vi "Stop Module.vi"(6 "Timeout to Wait for Stop (s) (-1: no timeout)":dbl=-1.0, 8 "error in":errorcluster, 9 "Wait for Module to Stop? (F)":bool, 10 "Origin":string) -> (0 "error out":errorcluster)   [LabVIEW 2025, in "CML UI.lvlib"]
doc: "Send the Stop request to the Module's Main.vi.\n\nIf <b>Wait for Module to Stop?</b> is TRUE, this VI will wait until the module main VI stops, and will timeout at the <b>Timeout to Wait for Stop</b> value. This value defaults to \"-1\", which means the VI will not timeout, and will always wait until the module main VI stops before completing execution.\n\nNote: The <b>Timeout to Wait for Stop</b> value is ignored if 'Wait for Module to Stop?' is set to FALSE.\n_____\nBased on DQMH Project Template 4.0.0.47.\n\n<b>Note:</b> This VI was modified by the <b>Validate DQMH Module</b> tool to add calls to the Semaphore VIs to synchronize actions between the Start Module and Stop Module VIs.\n_____\nBased on DQMH Dev Tools: Project Template 7.1.0.1503."
uses:
  CML UI.lvlib
  Stop Argument--cluster.ctl
  <vilib>/event_ctls.llb/usereventprio.ctl
panel:
  # "Note: The 'Timeout to Wait for Stop' value is ignored if 'Wait for Module to Stop?' is set to FALSE."
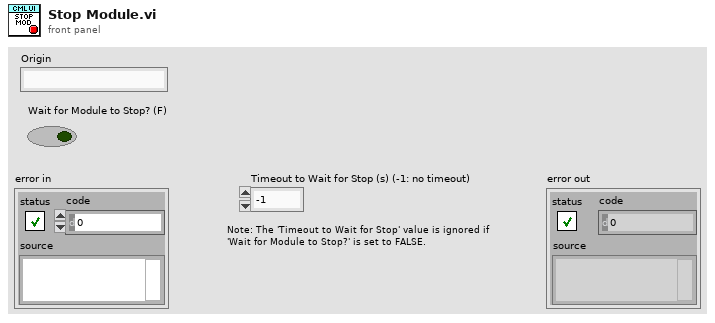
[diagram p1: front panel]
types:
  T1 = typedef "CML UI.lvlib/Stop Argument--cluster.ctl" = cluster{"Origin":string, "Exit via Stop Module Req?":bool, "Wait for Module to stop?":bool}
  T2 = typedef "usereventprio.ctl" = enum32{"high priority", "normal priority"}
  T3 = typedef "CML UI.lvlib/Request Events--cluster.ctl" = cluster{"Stop Module":refnum<user-event>, "Show Panel":refnum<user-event>, "Hide Panel":refnum<user-event>, "Get Module Execution Status":refnum<user-event>, "Show Diagram":refnum<user-event>}
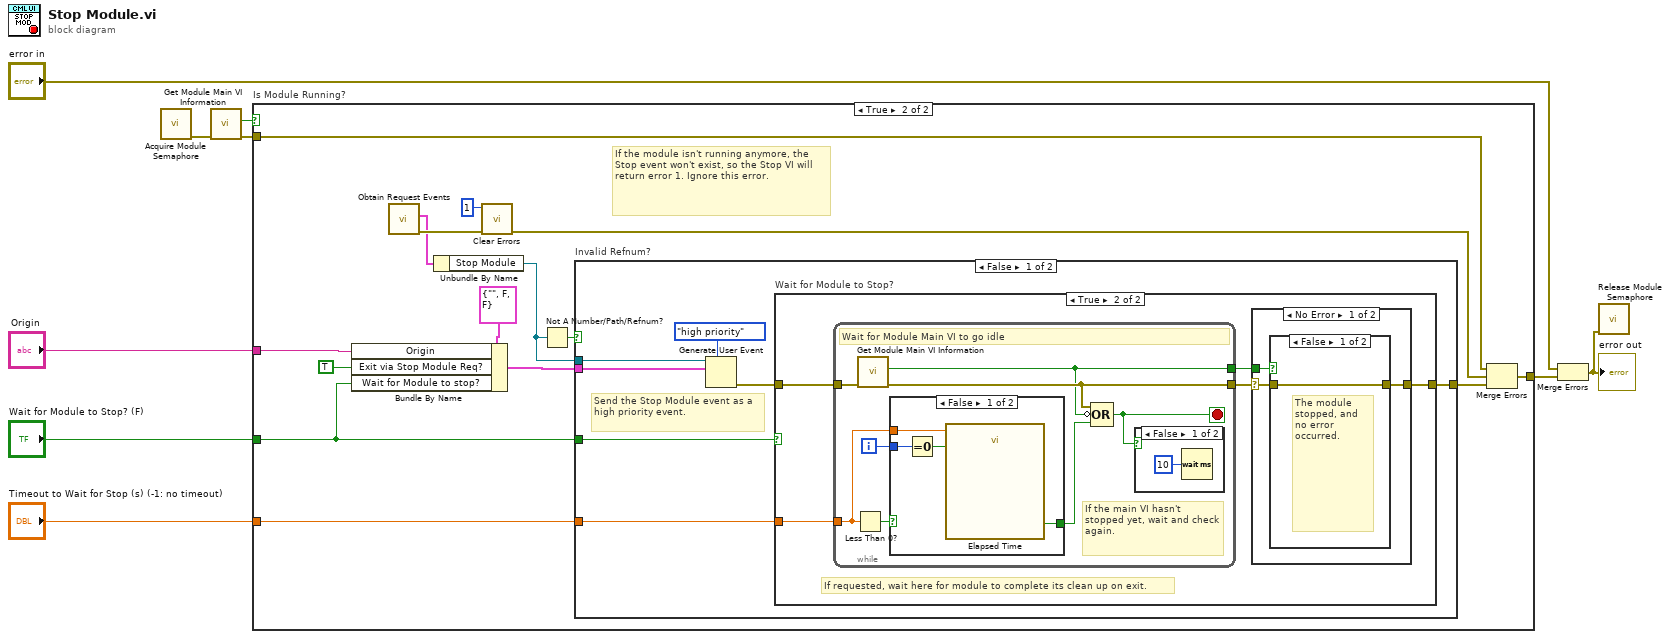
[diagram p0: block diagram]
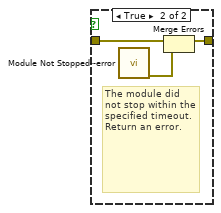
[diagram p4: hidden frame]
diagram:
  n1 = call "Acquire Module Semaphore.vi"() -> ("error out"=w1:errorcluster)  [unwired: 11 in]
  n2 = call "Get Module Main VI Information.vi"("error in"=w1) -> ("error out"=w6:errorcluster, "Is Module Running?"=w5:bool)  [unwired: 7 in, 2 out]
  n3 = case "Is Module Running?" shown="True" w5 {
    tunnel: [w10 w24] -> w9
    tunnel: "Origin" -> [_ w23]
    tunnel: w6 -> [w10 w15]
    tunnel: "Wait for Module to Stop? (F)" -> [_ w12]
    tunnel: "Timeout to Wait for Stop (s) (-1: no timeout)" -> [_ w11]
    frame False {
      # "The module is not running, there is no need to run the Stop Module code."
    }
    frame True {
      # "If the module isn't running anymore, the Stop event won't exist, so the Stop VI will return error 1. Ignore this error."
      n4 = Bundle By Name(cluster=T1 {"Origin"="", "Exit via Stop Module Req?"=FALSE, "Wait for Module to stop?"=FALSE} ("event data"), "Origin"=w23, "Exit via Stop Module Req?"=TRUE, "Wait for Module to stop?"=w12) -> (w18:T1)
      n5 = call "Obtain Request Events.vi"() -> ("error out"=w25:errorcluster, "CML UI Request Events"=w22:T3)  [unwired: 10 in]
      n6 = Unbundle By Name(w22) -> ("Stop Module"=w19:refnum<user-event>)
      n7 = call <vilib>:"Clear Errors.vi"("error in (no error)"=w25, "specific error code to clear (0: all)"=1) -> ("error out"=w14:errorcluster)  [unwired: 4 in, 1 out]
      n8 = Not A Number/Path/Refnum?(number/path/refnum=w19) -> (NaN/Path/Refnum?=w20:bool)
      n9 = case "Invalid Refnum?" shown="False" w20 {
        tunnel: [w27 _] -> w17
        tunnel: w19 -> [w32 _]
        tunnel: w18 -> [w30 _]
        tunnel: w12 -> [w28 _]
        tunnel: w11 -> [w26 _]
        frame False {
          # "Send the Stop Module event as a high priority event."
          n10 = Generate User Event(priority (normal)=usereventprio."high priority", user event=w32, event data cluster=w30) -> (error out=w29:errorcluster)  [unwired: 1 in, 1 out]
          n11 = case "Wait for Module to Stop?" shown="True" w28 {
            tunnel: w29 -> [w33 w37]
            tunnel: [w33 w35] -> w27
            tunnel: w26 -> [_ w38]
            frame False {
            }
            frame True {
              # "If requested, wait here for module to complete its clean up on exit."
              n12 = while {
                tunnel: w38 -> [w49]
                tunnel: w37 -> [w53]
                tunnel: [w52] -> w36
                tunnel: [w51] -> w34
                i -> [w54]
                stop <- w47 stop-if-true
                # "If the main VI hasn't stopped yet, wait and check again."
                # "Wait for Module Main VI to go idle"
                n13 = Less Than 0?(x=w49) -> (x < 0?=w48:bool)
                n14 = call "Get Module Main VI Information.vi"("error in"=w53) -> ("error out"=w52:errorcluster, "Is Module Running?"=w51:bool)  [unwired: 7 in, 2 out]
                n15 = case shown="False" w48 {
                  tunnel: w49 -> [w56 _]
                  tunnel: w54 -> [w58 _]
                  tunnel: [w57 _] -> w50
                  frame False {
                    n16 = Equal To 0?(x=w58) -> (x = 0?=w59:bool)
                    n17 = call "Elapsed Time"("Time Target (s)"=w56, "Reset"=w59) -> ("Time has Elapsed"=w57:bool)  [unwired: 10 in, 7 out]
                  }
                  frame True {
                    # "User specified a timeout of -1, so don't keep track of the elapsed time since this loop started."
                  }
                }
                n18 = Compound Arithmetic op=OR(w52, invert w51, w50) -> (w47:bool)
                n19 = case shown="False" w47 {
                  frame False {
                    n20 = Wait (ms)(milliseconds to wait=u32 10) -> ()  [unwired: 1 out]
                  }
                  frame True {
                  }
                }
              }
              n21 = case shown="No Error" w36 {
                selector: w36 -> [w40 w46]
                tunnel: [w39 w46] -> w35
                tunnel: w34 -> [w41 _]
                frame No Error {
                  n22 = case shown="False" w41 {
                    tunnel: w40 -> [w42 w45]
                    tunnel: [w42 w44] -> w39
                    frame False {
                      # "The module stopped, and no error occurred."
                    }
                    frame True {
                      # "The module did not stop within the specified timeout. Return an error."
                      n23 = call "Module Not Stopped--error.vi"() -> ("error out"=w43:errorcluster)  [unwired: 11 in]
                      n24 = Merge Errors(w45, w43) -> (w44:errorcluster)
                    }
                  }
                }
                frame Error {
                  # "An error occurred while waiting for the module to stop. Return that error."
                }
              }
            }
          }
        }
        frame True {
          # "Module is exiting. No need to send the standard \"not running\" error that is sent in other request VIs."
        }
      }
      n25 = Merge Errors(w15, w14, w17) -> (w24:errorcluster)
    }
  }
  n26 = Merge Errors("error in", w9) -> (w3:errorcluster)
  "error out" <- w3
  n27 = call "Release Module Semaphore.vi"("error in"=w3) -> ()  [unwired: 10 in, 1 out]
